vi "ToString.vi"(0 "reference in":refnum<class "G#Interface.lvclass">, 5 "error in (no error)":errorcluster) -> (14 "reference out":refnum<class "G#Interface.lvclass">, 15 "string":string, 19 "error out":errorcluster)   [LabVIEW 2020, in "G#Interface.lvclass"]
doc: "Defines a method that allows a class to return one string as a representation of the object."
uses:
  <vilib>/addons/_AddQ/G#Interface/G#Interface.lvclass
  <vilib>/addons/_AddQ/G#Interface/G#Interface.lvclass/G#Interface.ctl
  <vilib>/addons/_AddQ/G#Object/G#Object.lvclass
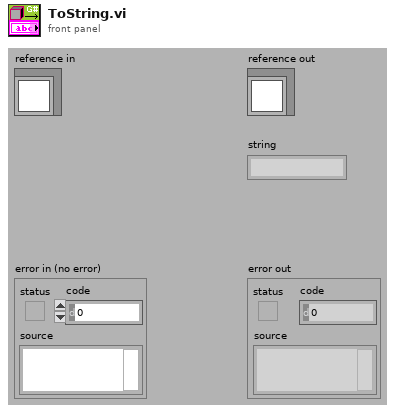
[diagram p1: front panel]
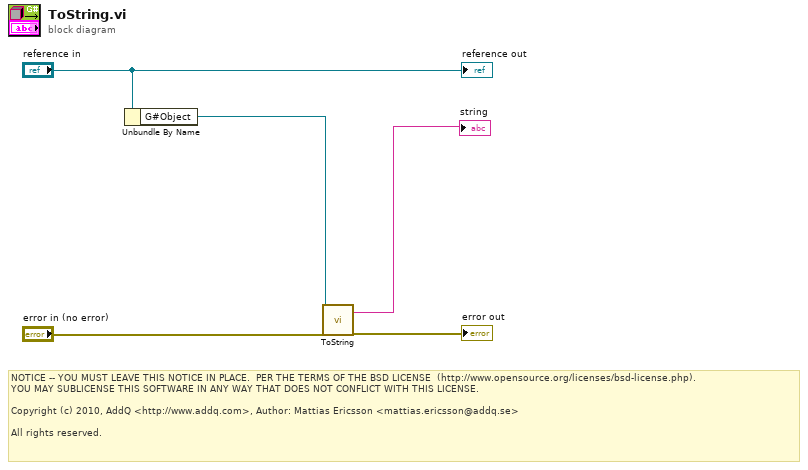
[diagram p0: block diagram]
diagram:
  # "NOTICE -- YOU MUST LEAVE THIS NOTICE IN PLACE.  PER THE TERMS OF THE BSD LICENSE  (http://www.opensource.org/licenses/bsd-license.php).\nYOU MAY SUBLICENSE THIS SOFTWARE IN ANY WAY THAT DOES NOT CONFLICT WITH THIS LICENSE.\n\nCopyright (c) 2010, AddQ <http://www.addq.com>, Author: Mattias Ericsson <mattias.ericsson@addq.se>\n\nAll rights reserved."
  n1 = Unbundle By Name("reference in") -> ("G#Object"=w3:refnum<class "G#Object.lvclass">)
  n2 = call-dynamic "ToString.vi"("reference in"=w3, "error in (no error)"="error in (no error)") -> ("string"=→"string":string, "error out"=→"error out":errorcluster)  [unwired: 15 in, 1 out]
  "reference out" <- "reference in"
